vi "RT Host.vi"() -> ()   [LabVIEW 2018]
uses:
  <vilib>/rvi/interface/nirviMethod/nirviMethod.xnode
  <vilib>/FPGAPlugInAG/Dynamic/niLvFpga_Run_Dynamic.vi
  <vilib>/FPGAPlugInAG/Dynamic/niLvFpga_AcknowledgeIrq_Dynamic.vi
  <vilib>/rvi/interface/nirviMethod/StockFPGA_InlinedMethodWaitForSingleIRQ.vi
  <vilib>/FPGAPlugInAG/Dynamic/niLvFpga_WaitOnIrq_Dynamic.vi
  <vilib>/rvi/interface/nirviCloseFPGA/nirviCloseFPGA.xnode
  <vilib>/FPGAPlugInAG/Dynamic/niLvFpga_Abort_Dynamic.vi
  <vilib>/rvi/interface/nirviOpenFPGA/nirviOpenFPGA.xnode
  <vilib>/FPGAPlugInAG/Dynamic/niLvFpga_Close_Dynamic.vi
  <vilib>/FPGAPlugInAG/Dynamic/niLvFpga_ReadFifo_Dynamic.vi
  <vilib>/rvi/errors/niLvFpgaMergeErrorWithErrorCode.vi
  <vilib>/FPGAPlugInAG/Dynamic/niLvFpga_WriteFifo_Dynamic.vi
  VS FPGA Addon CD Master LV2018/Source/Tests/System Tests/DMA Channels Basic Testing/Assets/DMA Channels cRIO FPGA Project/Bitfiles/cRIO 9039 FPGA Personality.lvbitx
  VS FPGA Addon CD Master LV2018/Source/Tests/System Tests/DMA Channels Basic Testing/Assets/DMA Channels cRIO FPGA Project/cRIO FPGA Personality.vi
  <vilib>/FPGAPlugInAG/cRIO-9039 (Sync)/niLvFpga_Open_cRIO-9039 (Sync).vi
  <vilib>/rvi/interface/common/dynamic/niFpgaDynamicAddResources.vi
panel:
  out "Waveform Graph 2":sgl[](graph)
  out "Waveform Graph 1":sgl[](graph)
  out "error out":errorcluster
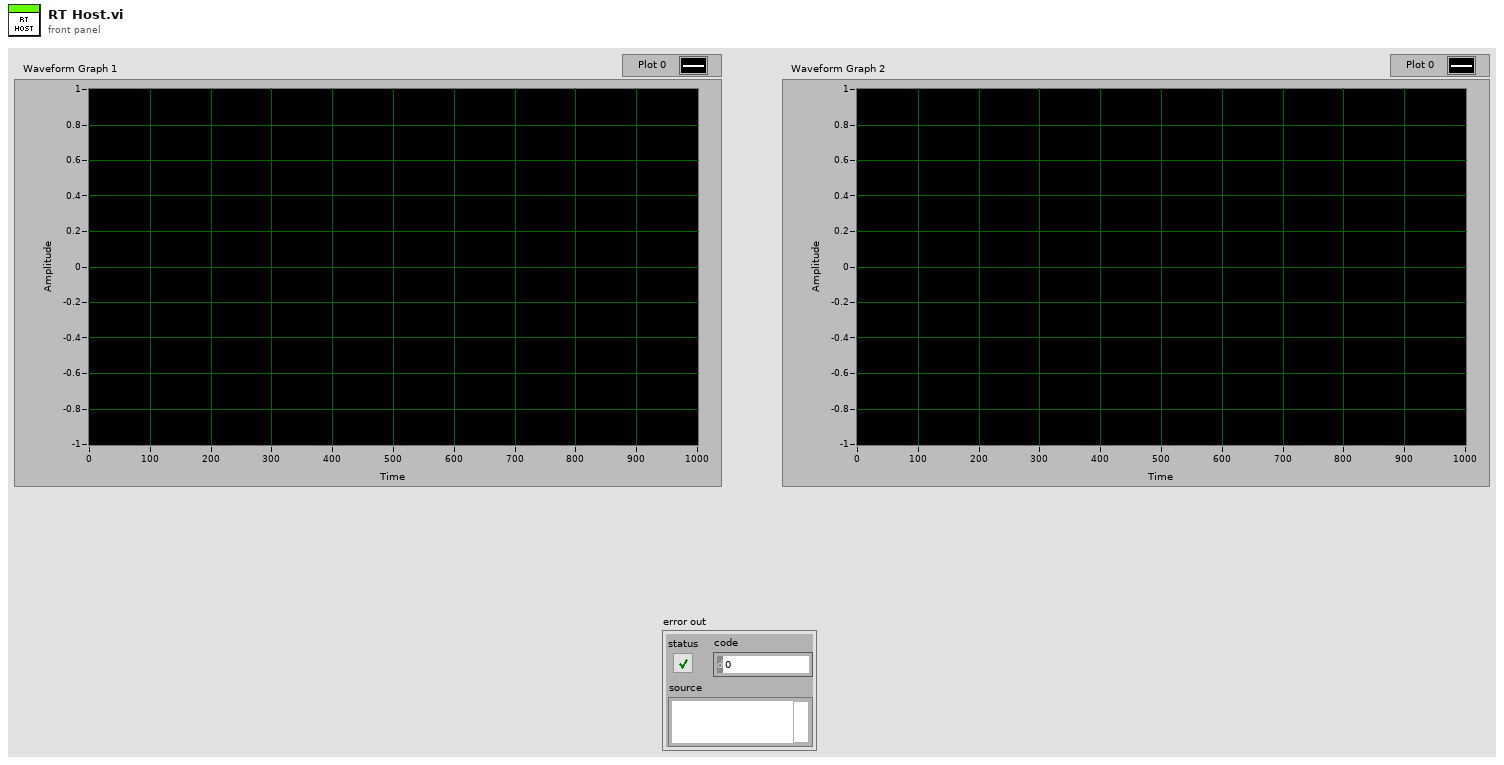
[diagram p1: front panel]
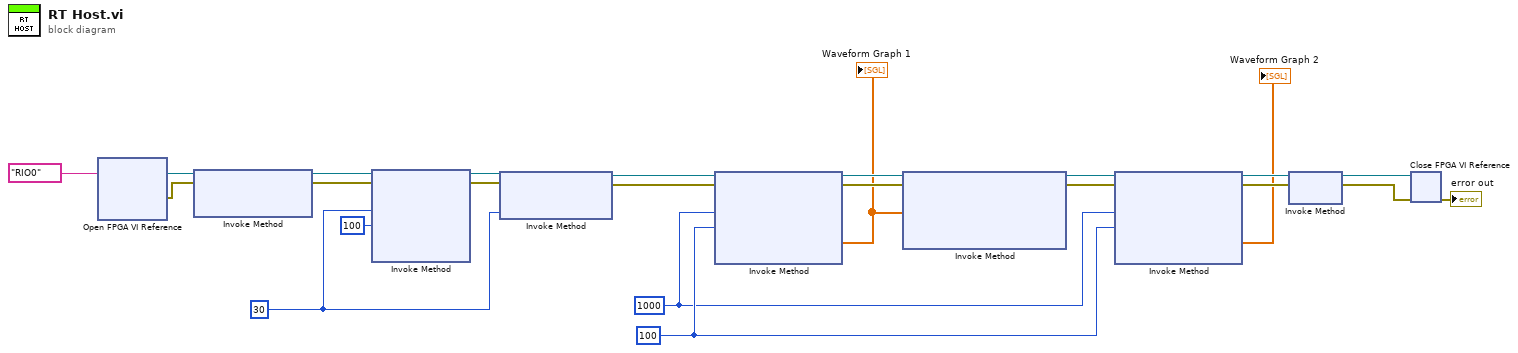
[diagram p0: block diagram]
diagram:
  w1 = u32 1000 ("Number of Elements")
  w2 = 100 ("Timeout (ms)")
  w22 = 30 ("IRQ Number(s)")
  n1 = xnode "Open FPGA VI Reference"("resource name"=tag "RIO0") -> ("FPGA VI Reference Out"=w13:refnum<k20>, "error out"=w11:errorcluster)  [unwired: 1 in]
  n2 = xnode "Invoke Method"("FPGA VI Reference In"=w13, "error in"=w11) -> ("FPGA VI Reference Out"=w24:refnum<k20>, "error out"=w23:errorcluster)  [unwired: 1 in]
  n3 = xnode "Invoke Method"("FPGA VI Reference In"=w24, "error in"=w23, "IRQ Number(s)"=w22, "Timeout (ms)"=100) -> ("FPGA VI Reference Out"=w21:refnum<k20>, "error out"=w20:errorcluster)  [unwired: 2 out]
  n4 = xnode "Invoke Method"("FPGA VI Reference In"=w21, "error in"=w20, "IRQ Number(s)"=w22) -> ("FPGA VI Reference Out"=w15:refnum<k20>, "error out"=w14:errorcluster)
  n5 = xnode "Invoke Method"("FPGA VI Reference In"=w15, "error in"=w14, "Number of Elements"=w1, "Timeout (ms)"=w2) -> ("FPGA VI Reference Out"=w10:refnum<k20>, "error out"=w9:errorcluster, "Data"=w8:sgl[])  [unwired: 1 out]
  "Waveform Graph 1" <- w8
  n6 = xnode "Invoke Method"("FPGA VI Reference In"=w10, "error in"=w9, "Data"=w8) -> ("FPGA VI Reference Out"=w7:refnum<k20>, "error out"=w6:errorcluster)  [unwired: 1 in, 1 out]
  n7 = xnode "Invoke Method"("FPGA VI Reference In"=w7, "error in"=w6, "Number of Elements"=w1, "Timeout (ms)"=w2) -> ("FPGA VI Reference Out"=w5:refnum<k20>, "error out"=w4:errorcluster, "Data"=→"Waveform Graph 2":sgl[])  [unwired: 1 out]
  n8 = xnode "Invoke Method"("FPGA VI Reference In"=w5, "error in"=w4) -> ("FPGA VI Reference Out"=w18:refnum<k20>, "error out"=w17:errorcluster)
  n9 = xnode "Close FPGA VI Reference"("FPGA VI Reference In"=w18, "error in"=w17) -> ("error out"=→"error out":errorcluster)
